vi "Write StdErr.vi"(8 "error in (no error)":errorcluster, 10 "StdErr":string, 11 "ParsedData in":refnum<class "ParsedData.lvclass">) -> (0 "error out":errorcluster, 3 "ParsedData out":refnum<class "ParsedData.lvclass">)   [LabVIEW 2022 SP3, in "ArgumentParser.lvlib" / "ParsedData.lvclass"]
uses:
  ParsedData.lvclass
  ParsedData.lvclass/ParsedData.ctl
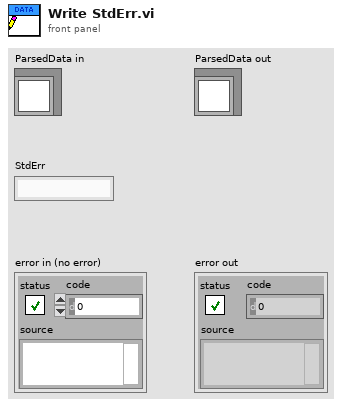
[diagram p1: front panel]
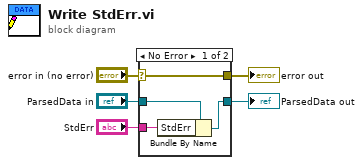
[diagram p0: block diagram]
diagram:
  n1 = case shown="No Error" "error in (no error)" {
    selector: "error in (no error)" -> [w9 w10]
    tunnel: [w9 w10] -> w4
    tunnel: [w7 w11] -> w2
    tunnel: "ParsedData in" -> [w8 w11]
    tunnel: "StdErr" -> [w6 _]
    frame No Error {
      n2 = Bundle By Name(cluster=w8, "StdErr"=w6) -> (w7:refnum<class "ParsedData.lvclass">)
    }
    frame Error {
    }
  }
  "error out" <- w4
  "ParsedData out" <- w2
